vi "Write Value to Property Key.vi"(8 "error in (no error)":errorcluster, 9 "Value":variant=variant(u32 1), 10 "Key":string, 11 "Service in":refnum<class "Service.lvclass">) -> (0 "error out":errorcluster, 3 "Service out":refnum<class "Service.lvclass">)   [LabVIEW 2024, in "Ramses Framework.lvlib" / "Service.lvclass"]
uses:
  Service.lvclass
  Service.lvclass/Service.ctl
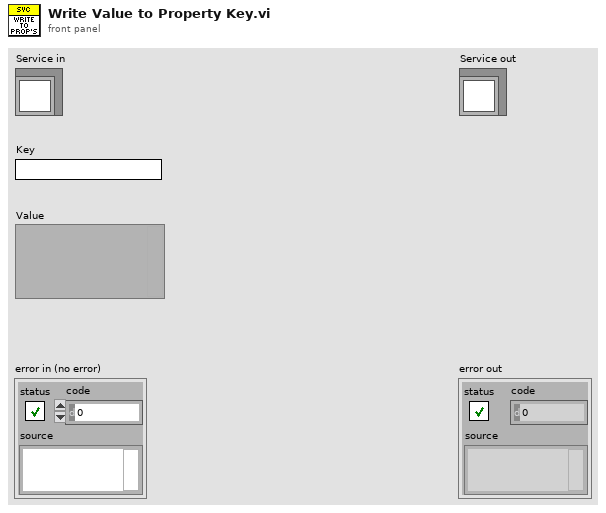
[diagram p1: front panel]
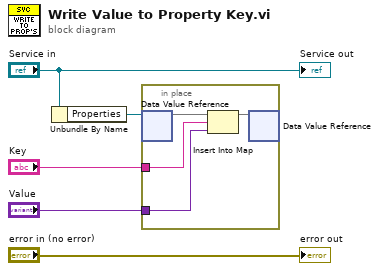
[diagram p0: block diagram]
diagram:
  n1 = Unbundle By Name("Service in") -> ("Properties"=w3:refnum<data-value>)
  n2 = in-place {
    in-place-border: "Value" -> [w6]
    in-place-border: "Key" -> [w7]
    n3 = in-place-dvr #1(w3) -> (w9:map{string, variant})  [unwired: 1 out]
    n4 = Insert Into Map(map in=w9, key=w7, value=w6) -> (map out=w8:map{string, variant})  [unwired: 2 out]
    n5 = in-place-dvr #1(w8) -> ()  [unwired: 2 out]
  }
  "error out" <- "error in (no error)"
  "Service out" <- "Service in"
